vi "ZLIB Open Unzip__ogtk.vi"   [LabVIEW 2020]
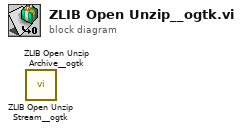
[diagram p0: block diagram]
diagram:
  n1 = call <userlib>:"ZLIB Open Unzip Stream__ogtk.vi"() -> ()  [unwired: 6 in, 2 out]
  n2 = call <userlib>:"ZLIB Open Unzip Archive__ogtk.vi"() -> ()  [unwired: 6 in, 2 out]
